vi "enumerate All Ports.vi"(8 "error in":errorcluster) -> (0 "error out":errorcluster)   [LabVIEW 2021, in "CycloneControlSDK.lvlib"]
doc: "extern \"C\" void _cdecl enumerateAllPorts(void);"
uses:
  CycloneControlSDK.lvlib
  CycloneControlSDK_64.dll
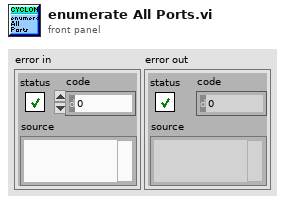
[diagram p1: front panel]
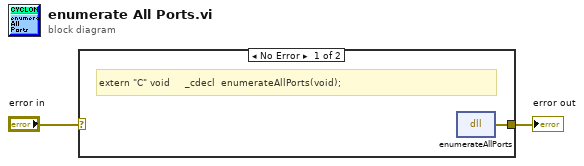
[diagram p0: block diagram]
diagram:
  n1 = case shown="No Error" "error in" {
    selector: "error in" -> [_ w4]
    tunnel: [w3 w4] -> w1
    frame No Error {
      # "extern \"C\" void     _cdecl  enumerateAllPorts(void);"
      n2 = dll-call lib="C:/PEMicro/cyclone/cycloneControl/controlsdk/examples/labview2018/user.lib/CycloneControlSDK/CycloneControlSDK_64.dll" fn="enumerateAllPorts"() -> (error out=w3:errorcluster)  [unwired: 4 in, 1 out]
    }
    frame Error {
    }
  }
  "error out" <- w1
